vi "ADCP_ES_Packet_To_Processed_Bytes.vi"(8 "error in (no error)":errorcluster, 10 "ES Packet In":T1, 11 "ADCP In":refnum<class "ADCP.lvclass">) -> (0 "error out":errorcluster, 2 "Processed Packet Bytes":u8[](array[numeric]), 3 "ADCP Out":refnum<class "ADCP.lvclass">)   [LabVIEW 2017, in "ADCP.lvclass"]
uses:
  ADCP.lvclass
  ADCP.lvclass/ADCP.ctl
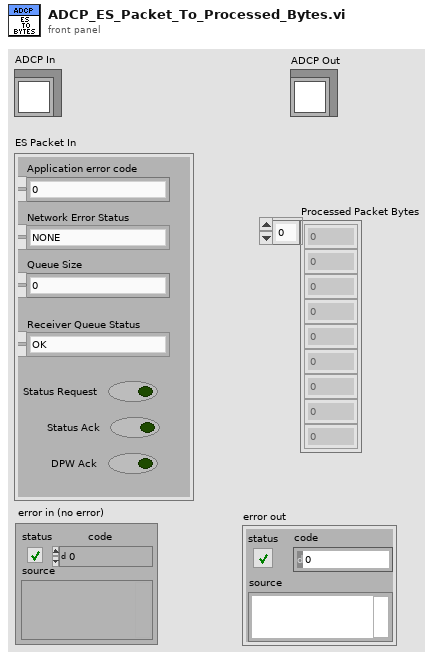
[diagram p1: front panel]
types:
  T1 = cluster{"Application error code":u16, "Network Error Status":enum16{"NONE", "CONNECTION_ALREADY_OPEN", "CONNECTION_ALREADY_CLOSED", "INVALID_FRAME_REQUEST"}, "Queue Size":u16, "Receiver Queue Status":enum16{"OK", "EMPTY", "FULL"}, "Status Request":bool, "Status Ack":bool, "DPW Ack":bool}
  T2 = enum16{"NONE", "CONNECTION_ALREADY_OPEN", "CONNECTION_ALREADY_CLOSED", "INVALID_FRAME_REQUEST"}
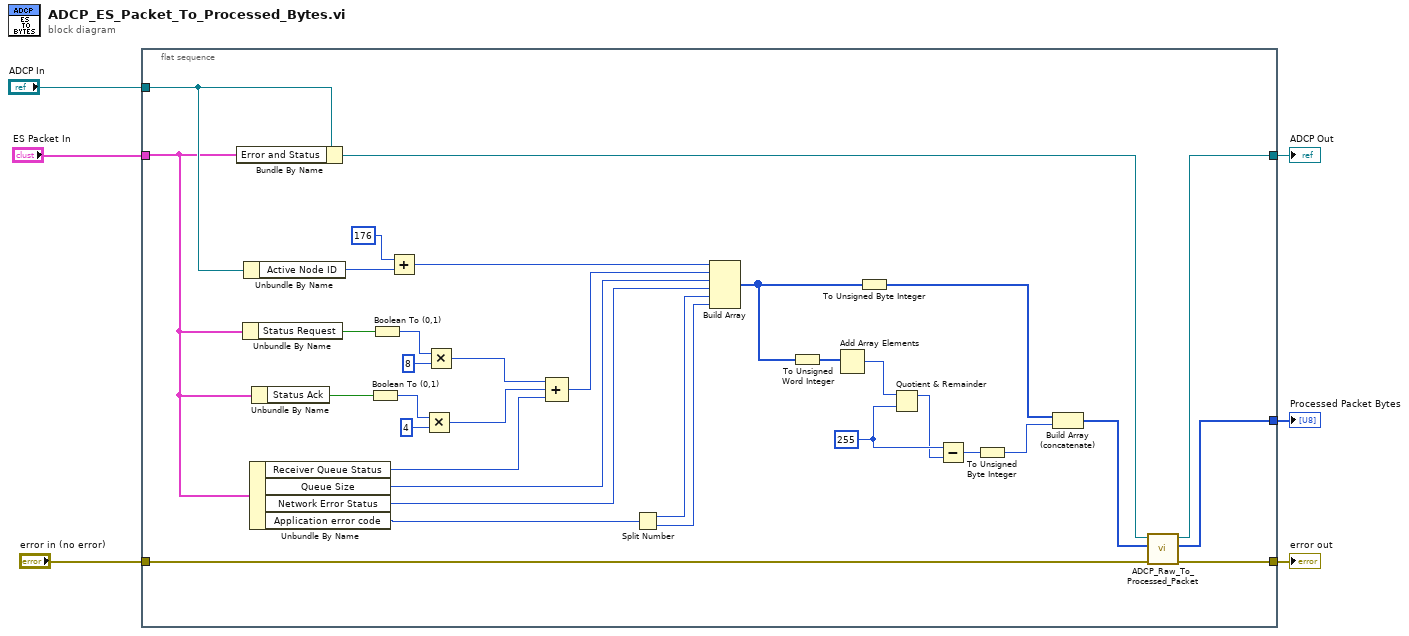
[diagram p0: block diagram]
diagram:
  n1 = flat-sequence {
    tunnel: "ADCP In" -> [w40]
    tunnel: "ES Packet In" -> [w31]
    tunnel: "error in (no error)" -> [w9]
    tunnel: [w10] -> w2
    tunnel: [w8] -> w3
    tunnel: [w11] -> w1
    frame #0 {
      w18 = u16 255 ("y")
      n2 = Bundle By Name(cluster=w40, "Error and Status"=w31) -> (w12:refnum<class "ADCP.lvclass">)
      n3 = Unbundle By Name(w31) -> ("Status Request"=w37:bool)
      n4 = Unbundle By Name(w40) -> ("Active Node ID"=w39:u8)
      n5 = Unbundle By Name(w31) -> ("Receiver Queue Status"=w28:enum16{"OK", "EMPTY", "FULL"}, "Queue Size"=w25:u16, "Network Error Status"=w24:T2, "Application error code"=w23:u16)
      n6 = Unbundle By Name(w31) -> ("Status Ack"=w34:bool)
      n7 = Boolean To (0,1)(Boolean=w34) -> (0, 1=w33:i16)
      n8 = Boolean To (0,1)(Boolean=w37) -> (0, 1=w36:i16)
      n9 = Add(x=u8 176, y=w39) -> (x+y=w27:u8)
      n10 = Multiply(x=w33, y=i16 4) -> (x*y=w29:i16)
      n11 = Multiply(x=w36, y=i16 8) -> (x*y=w30:i16)
      n12 = Compound Arithmetic op=ADD(w30, w29, w28) -> (w26:u16)
      n13 = Split Number(x=w23) -> (hi(x)=w22:u8, lo(x)=w21:u8)
      n14 = Build Array(w27, w26, w25, w24, w22, w21) -> (w15:u16[])
      n15 = To Unsigned Word Integer(number=w15) -> (unsigned 16bit integer=w20:u16[])
      n16 = Add Array Elements(numeric array=w20) -> (sum=w19:u16)
      n17 = To Unsigned Byte Integer(number=w15) -> (unsigned 8bit integer=w14:u8[])
      n18 = Quotient & Remainder(x=w19, y=w18) -> (x-y*floor(x/y)=w17:u16)  [unwired: 1 out]
      n19 = Subtract(x=w18, y=w17) -> (x-y=w16:u16)
      n20 = To Unsigned Byte Integer(number=w16) -> (unsigned 8bit integer=w7:u8)
      n21 = Build Array (concatenate)(w14, w7) -> (w13:u8[])
      n22 = call "ADCP_Raw_To_Processed_Packet.vi"("error in (no error)"=w9, "Raw Packet"=w13, "ADCP in"=w12) -> ("error out"=w8:errorcluster, "Processed Packet"=w10:u8[], "ADCP out"=w11:refnum<class "ADCP.lvclass">)  [unwired: 6 in]
    }
  }
  "error out" <- w3
  "Processed Packet Bytes" <- w2
  "ADCP Out" <- w1
